vi "Get_Bits_from_Reg.vi"(1 "Word Length":u16, 2 "Bit Number":i8, 3 "Reg Number":u16, 4 "Reg_in":u16[](array[numeric])) -> (0 "Bit Out":u16)   [LabVIEW 2011]
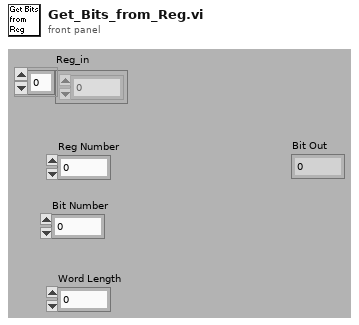
[diagram p1: front panel]
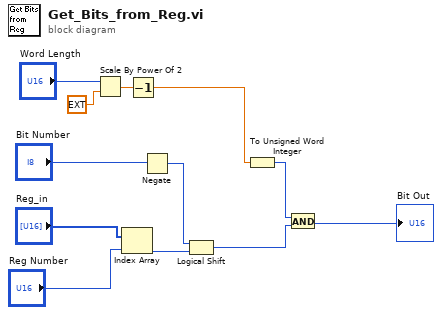
[diagram p0: block diagram]
diagram:
  n1 = Scale By Power Of 2(n="Word Length", x=ext 1.0) -> (x*2^n=w6:ext)
  n2 = Index Array(array="Reg_in", index="Reg Number") -> (element=w9:u16)
  n3 = Decrement(x=w6) -> (x-1=w4:ext)
  n4 = Negate(x="Bit Number") -> (-x=w2:i8)
  n5 = Logical Shift(y=w2, x=w9) -> (x << y=w8:u16)
  n6 = To Unsigned Word Integer(number=w4) -> (unsigned 16bit integer=w12:u16)
  n7 = And(x=w12, y=w8) -> (x .and. y?=→"Bit Out":u16)
